vi "Filter Panels.vi"(8 "error in (no error)":errorcluster, 10 "Panel Filter In":refnum<class "Panel Filter.lvclass">, 11 "2DArrayManager in":refnum<class "2DArrayManager.lvclass">) -> (0 "error out":errorcluster, 2 "Panel Filter":refnum<class "Panel Filter.lvclass">, 3 "2DArrayManager out":refnum<class "2DArrayManager.lvclass">)   [LabVIEW 2020, in "OOPanel.lvlib" / "2DArrayManager.lvclass"]
uses:
  2DArrayManager.lvclass
  Panel Filter/Panel Filter.lvclass
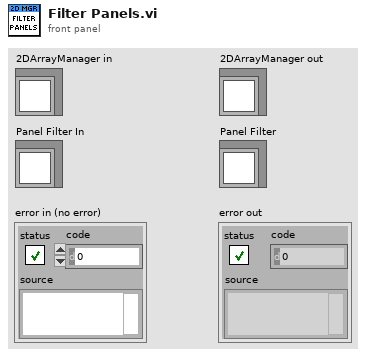
[diagram p1: front panel]
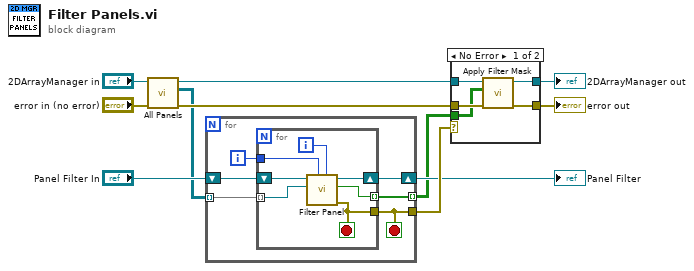
[diagram p0: block diagram]
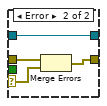
[diagram p2: hidden frame]
diagram:
  n1 = call "All Panels.vi"("error in (no error)"="error in (no error)", "2DArrayManager in"="2DArrayManager in") -> ("error out"=w10:errorcluster, "Panels"=w7:refnum<class "ArrayPanel.lvclass">[][], "2DArrayManager out"=w4:refnum<class "2DArrayManager.lvclass">)  [unwired: 7 in]
  n2 = for {
    shift-right: [w14] -> w6
    shift-left: "Panel Filter In" -> [w17]
    tunnel: w7 -> [w16] mode=indexing
    tunnel: [w13] -> w3 mode=indexing
    tunnel: [w12] -> w11
    i -> [w15]
    stop <- w12 stop-if-true
    n3 = for {
      shift-right: [w20] -> w14
      shift-left: w17 -> [w24]
      tunnel: w16 -> [w21] mode=indexing
      tunnel: w15 -> [w22]
      tunnel: [w19] -> w13 mode=indexing
      tunnel: [w18] -> w12
      i -> [w23]
      stop <- w18 stop-if-true
      n4 = call-dynamic "Filter Panel.vi"("Col"=w23, "Row"=w22, "Panel"=w21, "Panel Filter in"=w24) -> ("error out"=w18:errorcluster, "Include"=w19:bool, "Panel Filter out"=w20:refnum<class "Panel Filter.lvclass">)  [unwired: 5 in]
    }
  }
  "Panel Filter" <- w6
  n5 = case shown="No Error" w11 {
    selector: w11 -> [_ w30]
    tunnel: w4 -> [w29 w31]
    tunnel: w10 -> [w28 w33]
    tunnel: w3 -> [w27 _]
    tunnel: [w26 w31] -> w2
    tunnel: [w25 w32] -> w1
    frame No Error {
      n6 = call "Apply Filter Mask.vi"("error in (no error)"=w28, "Filter Mask"=w27, "2DArrayManager in"=w29) -> ("error out"=w25:errorcluster, "2DArrayManager out"=w26:refnum<class "2DArrayManager.lvclass">)  [unwired: 7 in]
    }
    frame Error {
      n7 = Merge Errors(w33, w30) -> (w32:errorcluster)
    }
  }
  "error out" <- w1
  "2DArrayManager out" <- w2
